vi "Cache File.vi"(8 "error in (no error)":errorcluster, 9 "Path":path, 10 "Response In":refnum<class "Response.lvclass">, 11 "Caching in":refnum<class "Caching.lvclass">) -> (0 "error out":errorcluster, 2 "Response":refnum<class "Response.lvclass">)   [LabVIEW 2020, in "HTTP Server.lvlib" / "Caching.lvclass"]
uses:
  Caching.lvclass
  Caching.lvclass/Caching.ctl
  <vilib>/IlluminatedG/IG HTTP Utils/HTTP Utils/Response/Response.lvclass
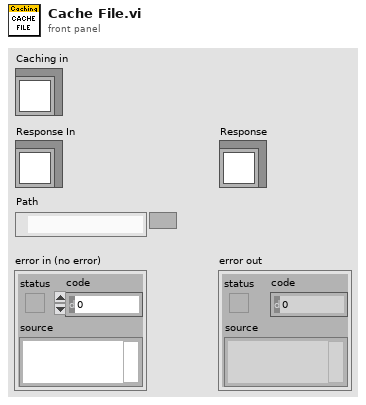
[diagram p1: front panel]
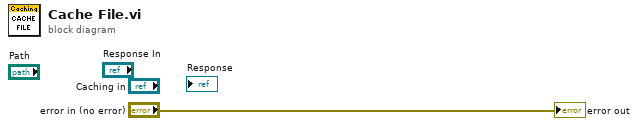
[diagram p0: block diagram]
diagram:
  "error out" <- "error in (no error)"
